vi "Convert Dual Tone Prop to String.vi"(8 "error in (no error)":errorcluster, 11 "dual tone properties":T1) -> (0 "error out":errorcluster, 3 "dual tone properties":string)   [LabVIEW 2021, in "AudioGenTypeDefs.lvlib"]
uses:
  AudioGenTypeDefs.lvlib
  dual tone properties.ctl
  dual tone types.ctl
  dual tone properties_JSON.ctl
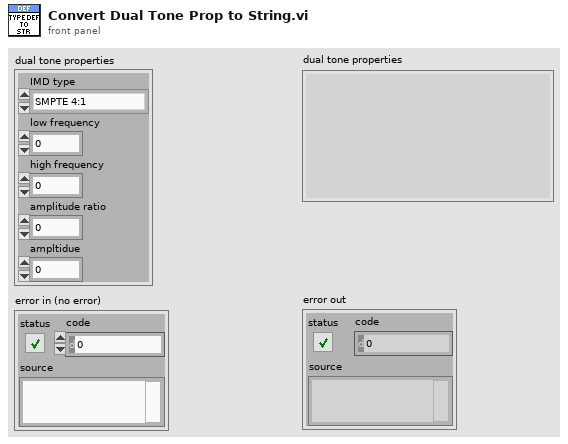
[diagram p1: front panel]
types:
  T1 = typedef "AudioGenTypeDefs.lvlib/dual tone properties.ctl" = cluster{"IMD type":T2, "low frequency":dbl, "high frequency":dbl, "amplitude ratio":dbl, "ampltidue":dbl}
  T2 = typedef "AudioGenTypeDefs.lvlib/dual tone types.ctl" = enum32{"SMPTE 4:1", "DIN", "CCIF 11k-12k", "CCIF 19k-20k", "Custom"}
  T3 = typedef "AudioGenTypeDefs.lvlib/dual tone properties_JSON.ctl" = cluster{"IMD standard":string, "low frequency":dbl, "high frequency":dbl, "amplitude ratio":dbl, "ampltidue":dbl}
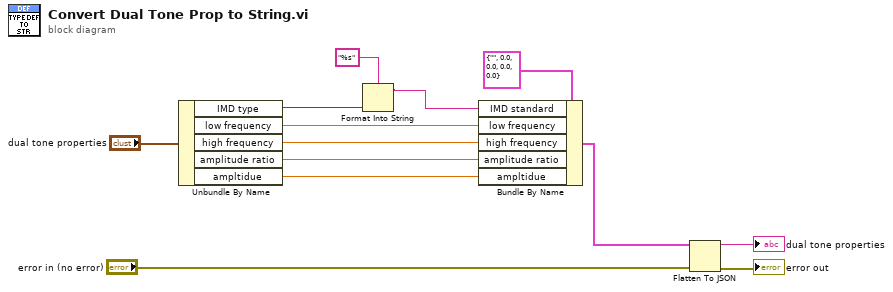
[diagram p0: block diagram]
diagram:
  n1 = Unbundle By Name("dual tone properties") -> ("IMD type"=w3:T2, "low frequency"=w7:dbl, "high frequency"=w6:dbl, "amplitude ratio"=w5:dbl, "ampltidue"=w4:dbl)
  n2 = Format Into String(format string="%s", w3) -> (resulting string=w1:string)  [unwired: 2 in, 1 out]
  n3 = Bundle By Name(cluster=T3 {"IMD standard"="", "low frequency"=0.0, "high frequency"=0.0, "amplitude ratio"=0.0, "ampltidue"=0.0} ("dual tone properties"), "IMD standard"=w1, "low frequency"=w7, "high frequency"=w6, "amplitude ratio"=w5, "ampltidue"=w4) -> (w12:T3)
  n4 = Flatten To JSON(anything=w12, error in (no error)="error in (no error)") -> (JSON string=→"dual tone properties":string, 11:→"error out":errorcluster)  [unwired: 1 in]
